vi "Logger.main.vi"(4 "Dir Path":path, 6 "#Channels":i32, 7 "Enum":T1, 8 "error in":errorcluster, 9 "TOAs":dbl[][](array[numeric]), 10 "RAW":i16[][](array[numeric])) -> (0 "error out":errorcluster)   [LabVIEW 2017]
uses:
  Logger.main.actions.ctl
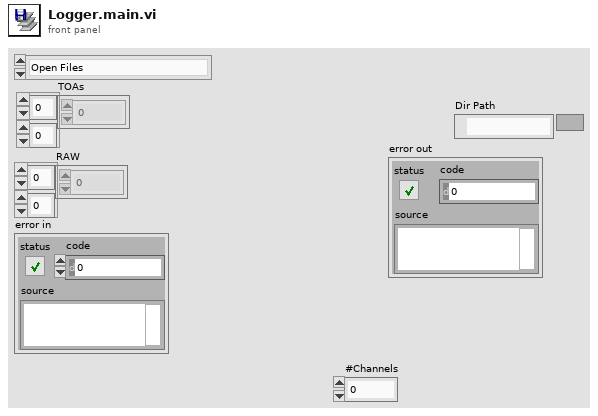
[diagram p1: front panel]
types:
  T1 = typedef "Logger.main.actions.ctl" = enum16{"Open Files", "Close Files", "WriteTOA", "WriteRAW"}
  T2 = enum16{"big-endian, network order", "native, host order", "little-endian"}
  T3 = enum16{"open", "replace", "create", "open or create", "replace or create", "replace or create with confirmation"}
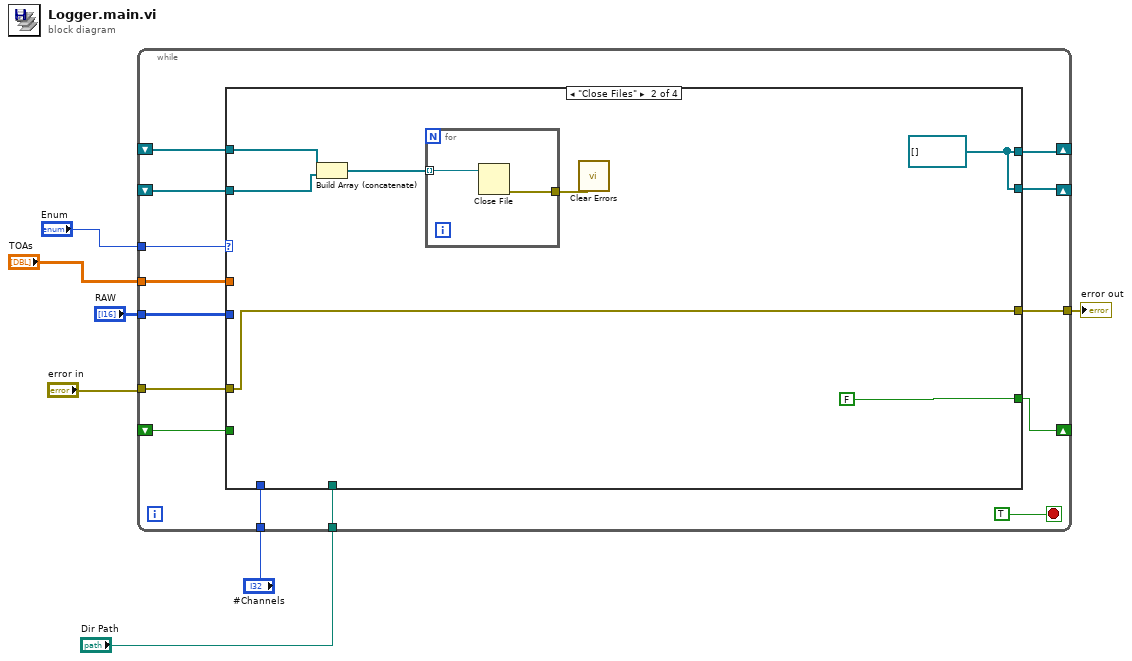
[diagram p0: block diagram]
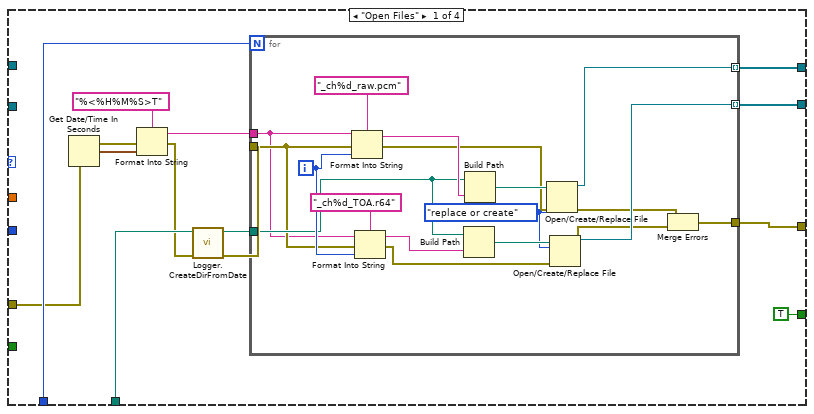
[diagram p2: hidden frame]
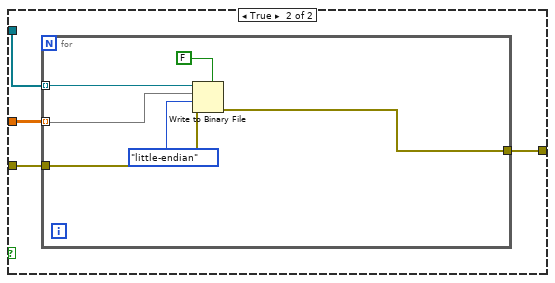
[diagram p4: hidden frame]
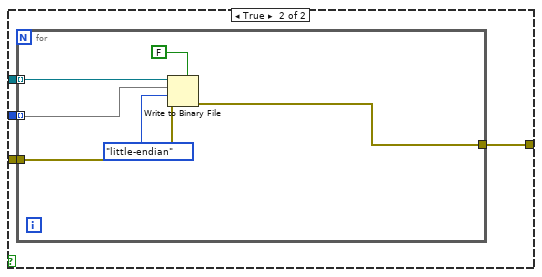
[diagram p6: hidden frame]
diagram:
  n1 = while {
    tunnel: "Enum" -> [w20]
    tunnel: "#Channels" -> [w19]
    tunnel: "Dir Path" -> [w18]
    shift-right: [w17] -> _
    shift-left: _ -> [w15]
    shift-right: [w16] -> _
    shift-left: _ -> [w14]
    tunnel: "TOAs" -> [w13]
    tunnel: "error in" -> [w12]
    tunnel: [w11] -> w1
    tunnel: "RAW" -> [w10]
    shift-right: [w9] -> _
    shift-left: _ -> [w8]
    stop <- TRUE stop-if-true
    n2 = case shown="\"Close Files\"" w20 {
      tunnel: w19 -> [w34 _ _ _]
      tunnel: w18 -> [w33 _ _ _]
      tunnel: [w26 w56 w67 w81] -> w17
      tunnel: [w25 w56 w65 w84] -> w16
      tunnel: w15 -> [_ w59 w67 w81]
      tunnel: w14 -> [_ w58 w65 w84]
      tunnel: w13 -> [_ _ w66 _]
      tunnel: w12 -> [w24 w54 w63 w82]
      tunnel: [w23 w54 w64 w83] -> w11
      tunnel: w10 -> [_ _ _ w80]
      tunnel: [TRUE FALSE w62 w79] -> w9
      tunnel: w8 -> [_ _ w62 w79]
      frame "Open Files" {
        n3 = Get Date/Time In Seconds() -> (seconds since 1Jan1904=w31:timestamp)
        n4 = Format Into String(format string="%<%H%M%S>T", error in=w24, w31) -> (resulting string=w29:string, error out=w28:errorcluster)  [unwired: 1 in]
        n5 = call "Logger.CreateDirFromDate.vi"("error in (no error)"=w28, "base path"=w33) -> ("error out"=w27:errorcluster, "Saving Dir"=w32:path)  [unwired: 8 in]
        n6 = for {
          N: w34 -> [_]
          tunnel: w32 -> [w49]
          tunnel: w29 -> [w35]
          tunnel: w27 -> [w43]
          tunnel: [w41] -> w26 mode=indexing
          tunnel: [w40] -> w25 mode=indexing
          tunnel: [w37] -> w23
          i -> [w51]
          w45 = T3."replace or create" ("operation (0:open)")
          n7 = Format Into String(format string="_ch%d_raw.pcm", initial string=w35, error in=w43, w51) -> (resulting string=w50:string, error out=w44:errorcluster)
          n8 = Format Into String(format string="_ch%d_TOA.r64", initial string=w35, error in=w43, w51) -> (resulting string=w48:string, error out=w42:errorcluster)
          n9 = Build Path(base path=w49, name or relative path=w48) -> (appended path=w46:path)
          n10 = Build Path(base path=w49, name or relative path=w50) -> (appended path=w47:path)
          n11 = Open/Create/Replace File(file path (use dialog)=w47, error in=w44, operation (0:open)=w45) -> (refnum out=w41:refnum<file>, error out=w39:errorcluster)  [unwired: 3 in, 1 out]
          n12 = Open/Create/Replace File(file path (use dialog)=w46, error in=w42, operation (0:open)=w45) -> (refnum out=w40:refnum<file>, error out=w38:errorcluster)  [unwired: 3 in, 1 out]
          n13 = Merge Errors(w39, w38) -> (w37:errorcluster)
        }
      }
      frame "Close Files" {
        w56 = refnum<file>[] []
        n14 = Build Array (concatenate)(w59, w58) -> (w57:refnum<file>[])
        n15 = for {
          tunnel: w57 -> [w61] mode=indexing
          tunnel: [w60] -> w55
          n16 = Close File(refnum=w61) -> (error out=w60:errorcluster)  [unwired: 1 in, 1 out]
        }
        n17 = call <vilib>:"Clear Errors.vi"("error in (no error)"=w55) -> ()  [unwired: 5 in, 2 out]
      }
      frame "WriteTOA" {
        n18 = case shown="False" w62 {
          tunnel: w66 -> [_ w72]
          tunnel: w65 -> [_ w71]
          tunnel: [w68 w70] -> w64
          tunnel: w63 -> [w68 w69]
          frame False {
          }
          frame True {
            n19 = for {
              tunnel: w72 -> [w76] mode=indexing
              tunnel: w71 -> [w77] mode=indexing
              tunnel: [w74] -> w70
              tunnel: w69 -> [w73]
              n20 = Write to Binary File(file (use dialog)=w77, data=w76, error in=w73, 5:FALSE ("prepend array or string size? (T)"), 9:T2."little-endian" ("byte order (0:big-endian, network order)")) -> (error out=w74:errorcluster)  [unwired: 1 in, 2 out]
            }
          }
        }
      }
      frame "WriteRAW" {
        n21 = case shown="False" w79 {
          tunnel: [w85 w89] -> w83
          tunnel: w82 -> [w85 w88]
          tunnel: w81 -> [_ w87]
          tunnel: w80 -> [_ w86]
          frame False {
          }
          frame True {
            n22 = for {
              tunnel: w86 -> [w93] mode=indexing
              tunnel: w87 -> [w94] mode=indexing
              tunnel: [w91] -> w89
              tunnel: w88 -> [w90]
              n23 = Write to Binary File(file (use dialog)=w94, data=w93, error in=w90, 5:FALSE ("prepend array or string size? (T)"), 9:T2."little-endian" ("byte order (0:big-endian, network order)")) -> (error out=w91:errorcluster)  [unwired: 1 in, 2 out]
            }
          }
        }
      }
    }
  }
  "error out" <- w1
